vi "ConfigUtilities - Update Selected Channels.vi"(8 "error in (no error)":errorcluster, 11 "Dependent Node Refs":T2[](array[typedef]) format="%.0x") -> (0 "error out":errorcluster, 1 "Val(Sgnl)":i32[](array[numeric]), 2 "Selected Channels":string[][](array[string]), 3 "Disabled Behavior":u8, 4 "Top Left Visible Cell":T1)   [LabVIEW 2016, in "UDP-Custom-Device System Explorer.lvlib"]
uses:
  UDP-Custom-Device System Explorer.lvlib
  <vilib>/NI Veristand/Custom Device API/Custom Device Item Ref.ctl
  <vilib>/Utility/miscctls.llb/LVRowAndColumnUnsignedTypeDef.ctl
  <vilib>/NI VeriStand/Custom Device API/Custom Device API.lvlib
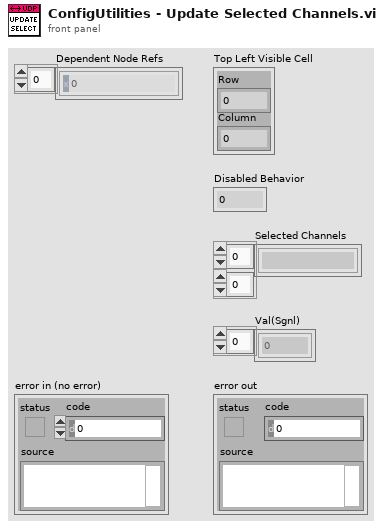
[diagram p1: front panel]
types:
  T1 = typedef "LVRowAndColumnUnsignedTypeDef.ctl" = cluster{"Row":u32, "Column":u32}
  T2 = typedef "Custom Device API.lvlib/Custom Device Item Ref.ctl" = u64
  T3 = typedef "Custom Device API.lvlib/Custom Device Item Info.ctl" = cluster{"Name":string, "Is Channel":bool, "GUID":string, "Is Waveform":bool}
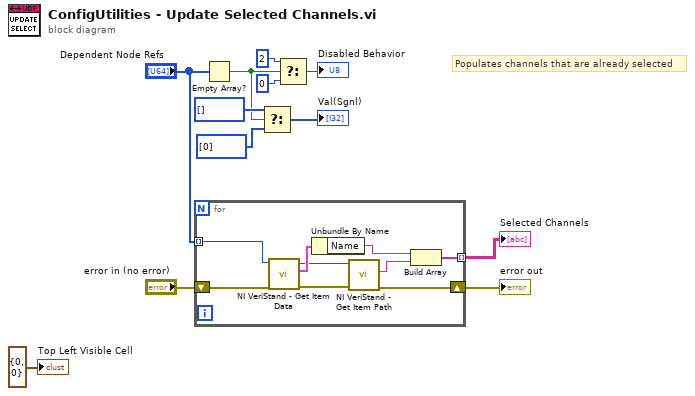
[diagram p0: block diagram]
diagram:
  # "Populates channels that are already selected"
  n1 = for {
    shift-right: [w21] -> w3
    shift-left: "error in (no error)" -> [w17]
    tunnel: "Dependent Node Refs" -> [w14] mode=indexing
    tunnel: [w19] -> w2 mode=indexing
    n2 = call <vilib>:"NI VeriStand - Get Item Data.vi"("error in (no error)"=w17, "Item Ref in"=w14) -> ("error out"=w16:errorcluster, "Item Info"=w18:T3, "Item Ref out"=w15:T2)  [unwired: 6 in, 1 out]
    n3 = Unbundle By Name(w18) -> ("Name"=w13:string)
    n4 = call <vilib>:"NI VeriStand - Get Item Path.vi"("error in (no error)"=w16, "Item Ref in"=w15) -> ("error out"=w21:errorcluster, "Path"=w20:string)  [unwired: 8 out]
    n5 = Build Array(w13, w20) -> (w19:string[])
  }
  "error out" <- w3
  "Selected Channels" <- w2
  n6 = Empty Array?(array="Dependent Node Refs") -> (empty?=w7:bool)
  n7 = Select(t=i32[] [] ("Value (Signaling)"), s=w7, f=i32[] [0]) -> (s? t:f=→"Val(Sgnl)":i32[])
  n8 = Select(t=u8 2, s=w7, f=u8 0) -> (s? t:f=→"Disabled Behavior":u8)
  "Top Left Visible Cell" <- T1 {"Row"=0, "Column"=0} ("Top Left Visible Cell")
